vi "Get Matrix - bitstream.vi"(6 "max dimensions (0: scalar)":i32, 8 "error in (no error)":errorcluster, 9 "data type":T2=enum."int", 10 "variable name":string, 11 "GOLPI ref. in":T3={"pipe handle"={"lv_proc.dll file path"=path "", "process instance handle"=[], "debug mode"=FALSE, "debug data"=[]}, "fast read timeout [ms]"=500, "fast read settle time [ms]"=10, "fast read to multiple [ms]"=1, "max elements per input line"=100, "slow read timeout [ms]"=5000, "stdin double format specifier"="%_16e", "max elements per stdout output column"=100, "console mode bitstream"=FALSE, "bitstream first read timeout [ms]"=1000, "bitstream read timeout [ms]"=50, "struct transfer possible"=FALSE, "matlab mode"=FALSE}) -> (0 "error out":errorcluster, 2 "data":T1, 3 "GOLPI ref. out":T3={"pipe handle"={"lv_proc.dll file path"=path "", "process instance handle"=[], "debug mode"=FALSE, "debug data"=[]}, "fast read timeout [ms]"=500, "fast read settle time [ms]"=10, "fast read to multiple [ms]"=1, "max elements per input line"=100, "slow read timeout [ms]"=5000, "stdin double format specifier"="%_16e", "max elements per stdout output column"=100, "console mode bitstream"=FALSE, "bitstream first read timeout [ms]"=1000, "bitstream read timeout [ms]"=50, "struct transfer possible"=FALSE, "matlab mode"=FALSE})   [LabVIEW 2020, in "GOLPI library.lvlib"]
doc: "Reads GNU Octave variable by means of bitstream via stdout.\nInput parameters are variable name, expected variable type (signed or unsigned integer, real, complex or string) and finally maximum dimensions count for the object, i.e. 0: scalars, 1: vector, 2: matrices. The function always returns 2D array of items. If the variable was vector it will be oriented as it was inside Octave. In case of strings matrix the data are returned as vector of strings. The integers are always returned as 64bit wide, reals and complex are always returned in double precission.\n'data type' is expected type of object to be transfered. 'real numeric' will transfer anything except complex and string."
uses:
  GOLPI library.lvlib
  GOLPI reference Type Def.ctl
  Pipe Handle.ctl
  Bitstream Data Type.ctl
  Bitstream Data.ctl
  Custom Error Codes Enum Type Def.vi
  LV Process library.lvlib
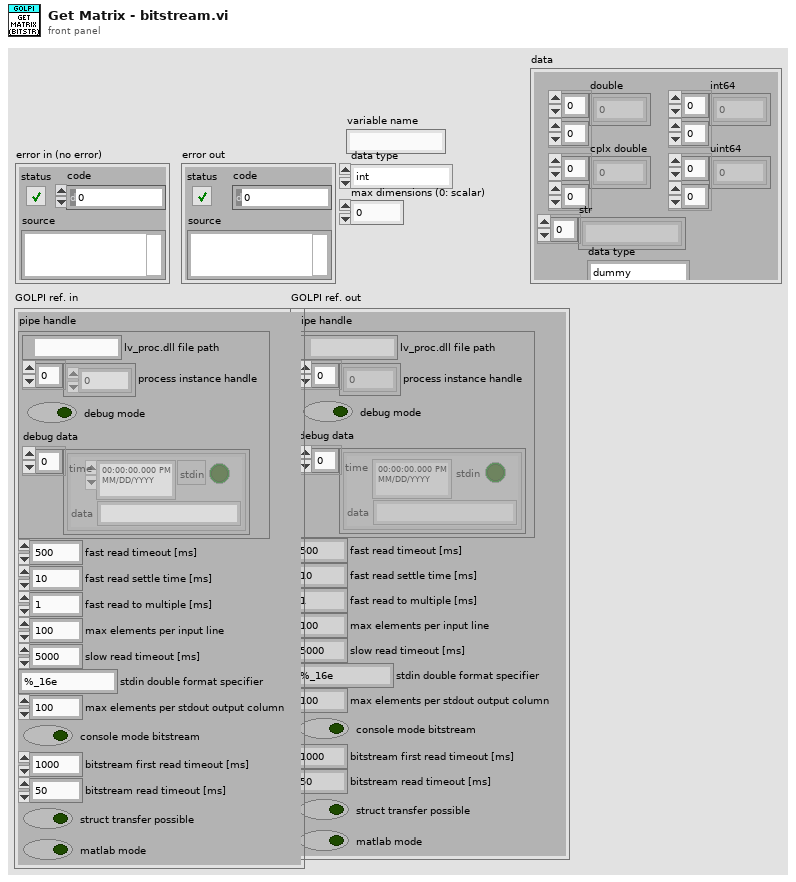
[diagram p1: front panel]
types:
  T1 = typedef "GOLPI library.lvlib/Bitstream Data.ctl" = cluster{"double":dbl[][], "cplx double":cdb[][], "int64":i64[][], "uint64":u64[][], "str":string[], "data type":T2}
  T2 = typedef "GOLPI library.lvlib/Bitstream Data Type.ctl" = enum16{"dummy", "int", "uint", "float", "complex", "str", "real numeric"}
  T3 = typedef "GOLPI library.lvlib/GOLPI reference Type Def.ctl" = cluster{"pipe handle":T4, "fast read timeout [ms]":u32, "fast read settle time [ms]":u32, "fast read to multiple [ms]":u32, "max elements per input line":u32, "slow read timeout [ms]":u32, "stdin double format specifier":string, "max elements per stdout output column":u32, "console mode bitstream":bool, "bitstream first read timeout [ms]":u32, "bitstream read timeout [ms]":u32, "struct transfer possible":bool, "matlab mode":bool}
  T4 = typedef "LV Process library.lvlib/Pipe Handle.ctl" = cluster{"lv_proc.dll file path":path, "process instance handle":u32[], "debug mode":bool, "debug data":cluster{"time":timestamp, "stdin":bool, "data":string}[]}
  T5 = typedef "GOLPI library.lvlib/Custom Error Codes Enum Type Def.vi" = enum16{"no error", "00 working directory PAR1 missing", "01 octave binary PAR1 missing", "02 octave report error PAR1", "03 empty output last cmd PAR1", "04 missing temporary file PAR1", "05 pwd PAR 1 not exist", "06 oct package not installed", "07 octave default binary missing", "10 var PAR1 not string, vect", "11 var PAR1 not num, scal, ~compl", "12 var PAR1 not num, scal, compl", "13 var PAR1 not num, vect, ~compl", "14 var PAR1 not num, vect, compl", "15 var PAR1 not num, mat, ~compl", "16 var PAR1 not num, mat, ~compl", "30 read timeout", "60 bitstream transport failed", "61 bitstream decode error PAR1", "62 bitstream cannot be set", "70 struct transfer not possible", "80 struct: cluster elem. PAR1 not implem.", "81 struct: structure field PAR1 not implem.", "82 struct: size mismatch of PAR1", "83 struct: type mismatch of PAR1", "98 internal error", "99 not finished", "90 Not supported in Matlab mode", "91 Matlab variable transfer error", "92 Matlab Script Error"}
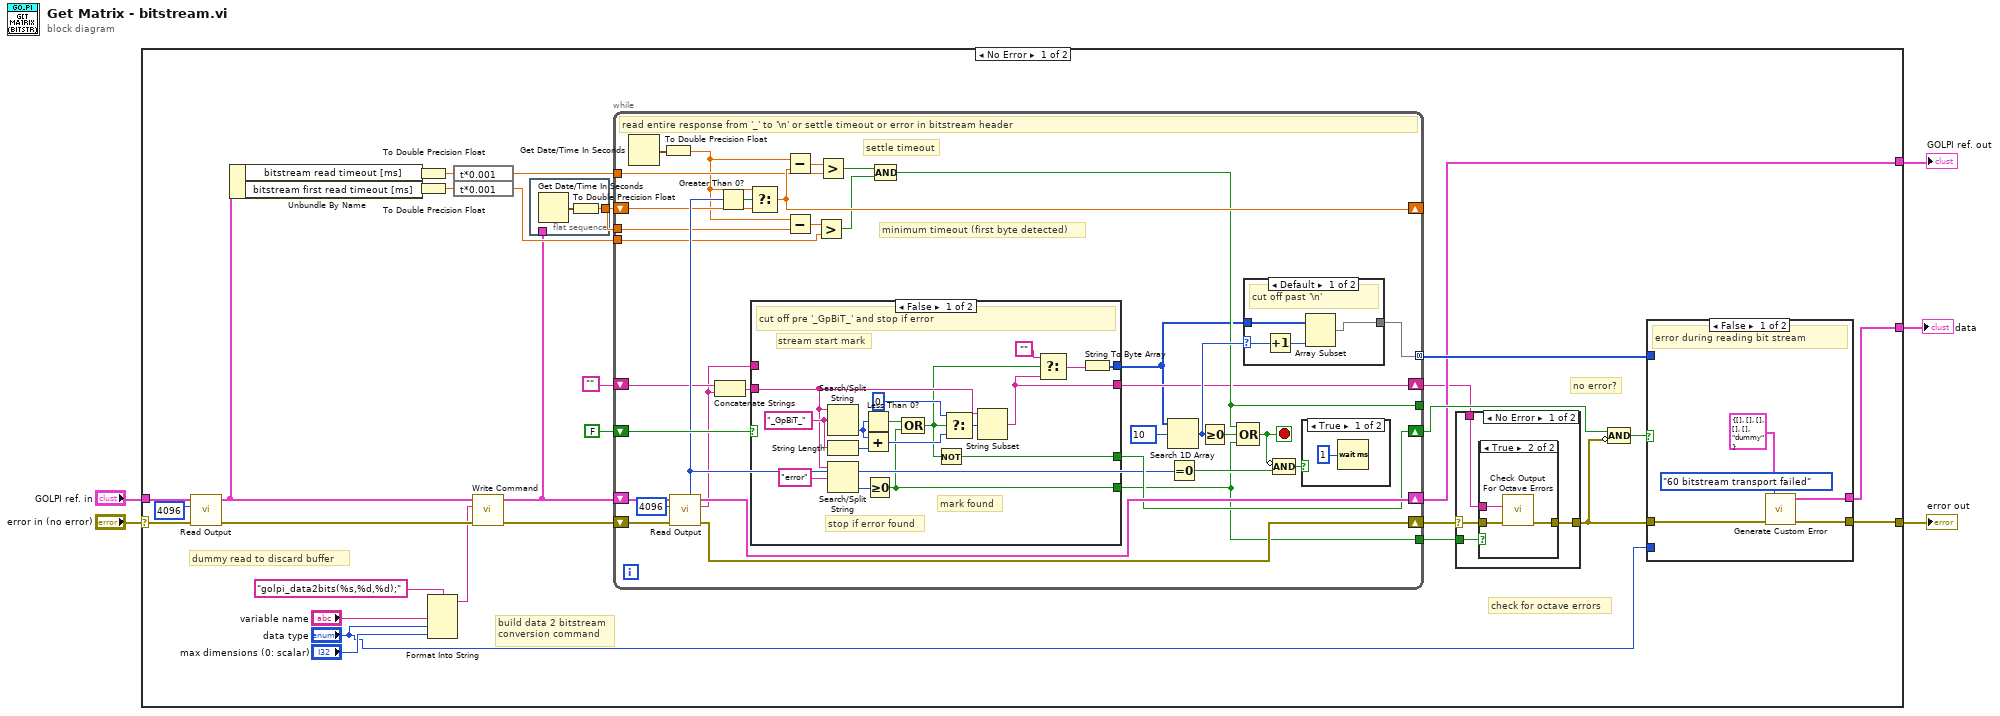
[diagram p0: block diagram]
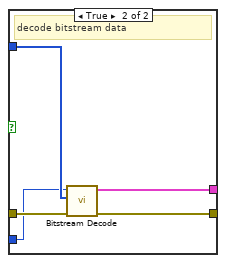
[diagram p2: hidden frame]
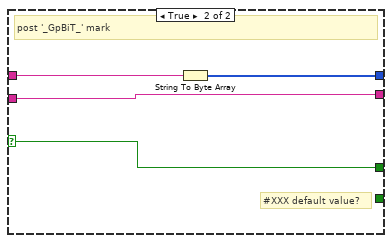
[diagram p5: hidden frame]
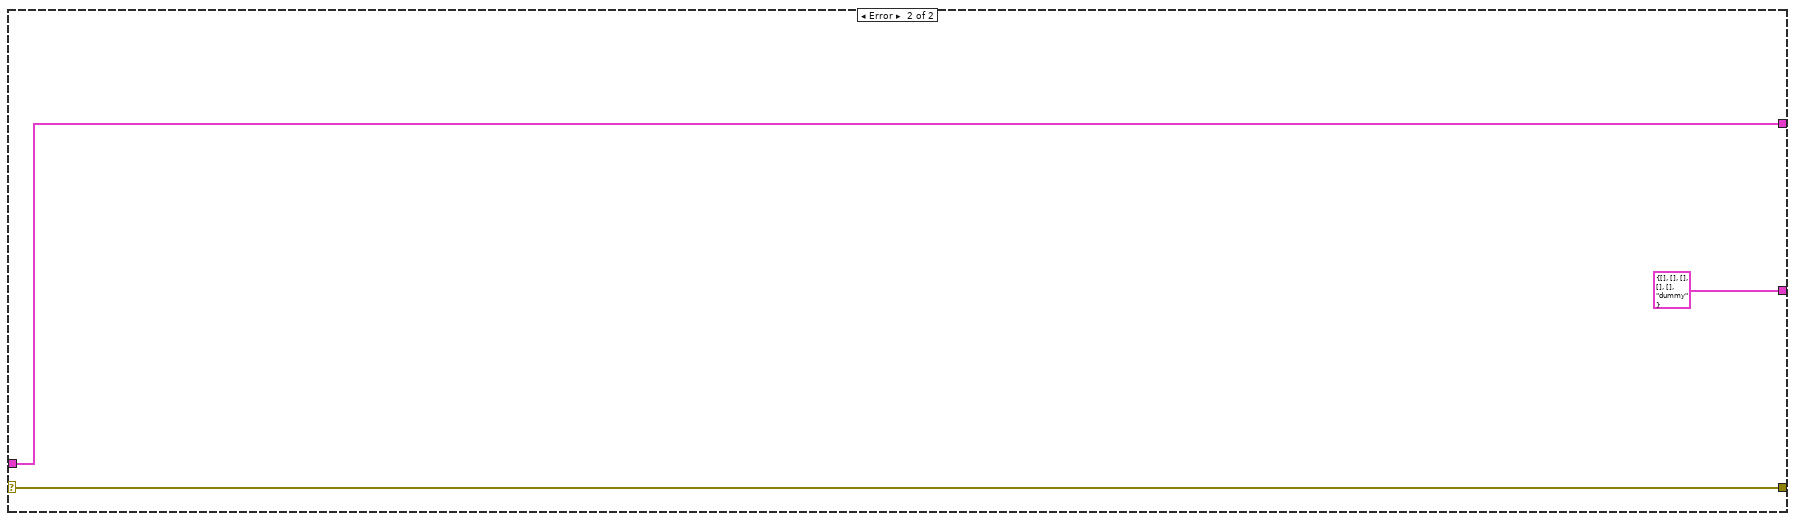
[diagram p8: hidden frame]
diagram:
  n1 = case shown="No Error" "error in (no error)" {
    selector: "error in (no error)" -> [w30 w120]
    tunnel: "GOLPI ref. in" -> [w27 w119]
    tunnel: [w32 w120] -> w5
    tunnel: [w14 w119] -> w2
    tunnel: [w23 T1 {"double"=[], "cplx double"=[], "int64"=[], "uint64"=[], "str"=[], "data type"=enum."dummy"} ("Cluster")] -> w1
    frame No Error {
      # "dummy read to discard buffer"
      # "check for octave errors"
      # "no error?"
      # "build data 2 bitstream\nconversion command"
      # "if octave not reported error"
      n2 = call "Read Output.vi"("error in"=w30, "byte count"=4096, "GOLPI ref. in"=w27) -> ("error out"=w29:errorcluster, "GOLPI ref. out"=w28:T3)  [unwired: 5 in, 2 out]
      n3 = Unbundle By Name(w28) -> ("bitstream read timeout [ms]"=w34:u32, "bitstream first read timeout [ms]"=w22:u32)
      n4 = To Double Precision Float(number=w34) -> (double precision float=w24:dbl)
      n5 = To Double Precision Float(number=w22) -> (double precision float=w20:dbl)
      n6 = Format Into String(format string="golpi_data2bits(%s,%d,%d);" ("initial string"), "variable name", "data type", "max dimensions (0: scalar)") -> (resulting string=w18:string)  [unwired: 2 in, 1 out]
      n7 = expression code="t*0.001"(w24) -> (w25:dbl)
      n8 = expression code="t*0.001"(w20) -> (w9:dbl)
      n9 = call "Write Command.vi"("error in"=w29, "command"=w18, "GOLPI ref. in"=w28) -> ("error out"=w35:errorcluster, "GOLPI ref. out"=w8:T3)  [unwired: 7 in]
      n10 = flat-sequence {
        tunnel: [w46] -> w21
        tunnel: w8 -> [_]
        frame #0 {
          n11 = Get Date/Time In Seconds() -> (seconds since 1Jan1904=w47:timestamp)
          n12 = To Double Precision Float(number=w47) -> (double precision float=w46:dbl)
        }
      }
      n13 = while {
        shift-right: [w86] -> w13
        shift-left: w35 -> [w90]
        shift-right: [w87] -> w14
        shift-left: w8 -> [w89]
        tunnel: [w77] -> w31 mode=concatenating
        tunnel: [w64] -> _
        shift-right: [w75] -> w33
        shift-left: FALSE -> [w76]
        shift-right: [w71] -> _
        shift-left: w21 -> [w72]
        tunnel: w25 -> [w70]
        tunnel: w21 -> [w69]
        tunnel: w9 -> [w67]
        shift-right: [w61] -> w10
        shift-left: "" -> [w63]
        tunnel: [w58] -> w11
        stop <- w79 stop-if-true
        # "minimum timeout (first byte detected)"
        # "settle timeout"
        # "read entire response from '_' to '\\n' or settle timeout or error in bitstream header"
        n14 = Get Date/Time In Seconds() -> (seconds since 1Jan1904=w82:timestamp)
        n15 = To Double Precision Float(number=w82) -> (double precision float=w57:dbl)
        n16 = call "Read Output.vi"("error in"=w90, "byte count"=4096, "GOLPI ref. in"=w89) -> ("error out"=w86:errorcluster, "read buffer"=w60:string, "GOLPI ref. out"=w87:T3, "bytes remaining"=w74:i32)  [unwired: 5 in]
        n17 = Concatenate Strings(w63, w60) -> (w62:string)
        n18 = Greater Than 0?(x=w74) -> (x > 0?=w73:bool)
        n19 = Select(t=w57, s=w73, f=w72) -> (s? t:f=w71:dbl)
        n20 = case shown="False" w76 {
          selector: w76 -> [_ w111]
          tunnel: [w98 w111] -> w75
          tunnel: w62 -> [w100 w110]
          tunnel: [w95 _] -> w58
          tunnel: [w91 w110] -> w61
          tunnel: [w97 w109] -> w59
          tunnel: w60 -> [_ w108]
          frame False {
            w107 = "_GpBiT_" ("search string/char (-)")
            # "stream start mark"
            # "mark found"
            # "stop if error found"
            # "cut off pre '_GpBiT_' and stop if error"
            n21 = Search/Split String(string=w100, search string/char (-)=w107) -> (offset of match=w105:i32)  [unwired: 1 in, 2 out]
            n22 = String Length(string=w107) -> (length=w106:i32)
            n23 = Search/Split String(string=w100, search string/char (-)="error") -> (offset of match=w102:i32)  [unwired: 1 in, 2 out]
            n24 = Less Than 0?(x=w105) -> (x < 0?=w96:bool)
            n25 = Add(x=w105, y=w106) -> (x+y=w104:i32)
            n26 = Greater Or Equal To 0?(x=w102) -> (x >= 0?=w95:bool)
            n27 = Compound Arithmetic op=OR(w96, w95) -> (w93:bool)
            n28 = Not(x=w93) -> (.not. x?=w98:bool)
            n29 = Select(t=0 ("byte count"), s=w93, f=w104) -> (s? t:f=w101:i32)
            n30 = String Subset(string=w100, offset (0)=w101) -> (substring=w91:string)  [unwired: 1 in]
            n31 = Select(t="", s=w93, f=w91) -> (s? t:f=w94:string)
            n32 = String To Byte Array(string=w94) -> (unsigned byte array=w97:u8[])
          }
          frame True {
            # "#XXX default value?"
            # "post '_GpBiT_' mark"
            n33 = String To Byte Array(string=w108) -> (unsigned byte array=w109:u8[])
          }
        }
        n34 = Subtract(x=w57, y=w71) -> (x-y=w81:dbl)
        n35 = Subtract(x=w57, y=w69) -> (x-y=w68:dbl)
        n36 = Greater?(x=w68, y=w67) -> (0:w66:bool)
        n37 = Greater?(x=w81, y=w70) -> (0:w65:bool)
        n38 = Compound Arithmetic op=AND(w65, w66) -> (w64:bool)
        n39 = Search 1D Array(1D array=w59, element=u8 10) -> (index of element=w78:i32)  [unwired: 1 in]
        n40 = Equal To 0?(x=w74) -> (x = 0?=w84:bool)
        n41 = Greater Or Equal To 0?(x=w78) -> (x >= 0?=w80:bool)
        n42 = Compound Arithmetic op=OR(w64, w80, w58) -> (w79:bool)
        n43 = case shown="Default" w78 {
          selector: w78 -> [w114 _]
          tunnel: w59 -> [w115 w116]
          tunnel: [w112 w116] -> w77
          frame Default {
            # "cut off past '\\n'"
            n44 = Increment(x=w114) -> (x+1=w113:i32)
            n45 = Array Subset(array=w115, length=w113) -> (w112:u8[])  [unwired: 1 in]
          }
          frame -1 {
          }
        }
        n46 = Compound Arithmetic op=AND(invert w79, w84) -> (w83:bool)
        n47 = case shown="True" w83 {
          frame True {
            n48 = Wait (ms)(milliseconds to wait=u32 1) -> ()  [unwired: 1 out]
          }
          frame False {
          }
        }
      }
      n49 = case shown="No Error" w13 {
        selector: w13 -> [w51 w56]
        tunnel: [w50 w56] -> w12
        tunnel: w11 -> [w49 _]
        tunnel: w10 -> [w48 _]
        frame No Error {
          n50 = case shown="True" w49 {
            tunnel: w51 -> [w52 w55]
            tunnel: [w52 w54] -> w50
            tunnel: w48 -> [_ w53]
            frame False {
            }
            frame True {
              n51 = call "Check Output For Octave Errors.vi"("error in"=w55, "read buffer"=w53) -> ("error out"=w54:errorcluster)  [unwired: 9 in]
            }
          }
        }
        frame Error {
        }
      }
      n52 = Compound Arithmetic op=AND(w33, invert w12) -> (w6:bool)
      n53 = case shown="False" w6 {
        tunnel: [w38 w45] -> w32
        tunnel: w31 -> [_ w44]
        tunnel: [T1 {"double"=[], "cplx double"=[], "int64"=[], "uint64"=[], "str"=[], "data type"=enum."dummy"} ("Cluster") w43] -> w23
        tunnel: w12 -> [w39 w42]
        tunnel: "data type" -> [_ w41]
        frame False {
          # "error during reading bit stream"
          n54 = call "Generate Custom Error.vi"("error in"=w39, "GOLPI error"=Custom_Error_Codes_Enum_Type_Def.vi."60 bitstream transport failed") -> ("error out"=w38:errorcluster)  [unwired: 9 in]
        }
        frame True {
          # "decode bitstream data"
          n55 = call "Bitstream Decode.vi"("error in (no error)"=w42, "bitstream"=w44, "data type"=w41) -> ("error out"=w45:errorcluster, "Cluster"=w43:T1)  [unwired: 7 in]
        }
      }
    }
    frame Error {
    }
  }
  "error out" <- w5
  "GOLPI ref. out" <- w2
  "data" <- w1
